vi "Write Horizontal Scrollbar.vi"(5 "Horizontal Scrollbar":bool, 9 "String in":refnum<class "String.lvclass">) -> (3 "String out":refnum<class "String.lvclass">)   [LabVIEW 2014, in "Raspberry Pi Compatible Compiler for LabVIEW.lvlib" / "String.lvclass"]
uses:
  String.lvclass
  String.lvclass/String.ctl
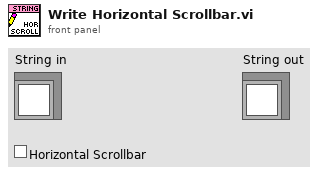
[diagram p1: front panel]
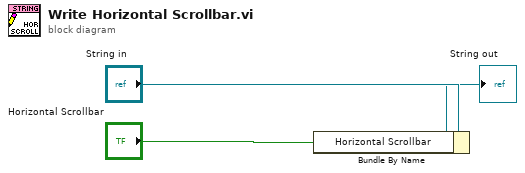
[diagram p0: block diagram]
diagram:
  n1 = Bundle By Name(cluster="String in", "Horizontal Scrollbar"="Horizontal Scrollbar") -> (→"String out":refnum<class "String.lvclass">)
